vi "Convert From Subpanel Tag.vi"(8 "error in":errorcluster, 11 "subpanel tag":string) -> (0 "error out":errorcluster, 1 "valid?":bool, 2 "subpanel UID":i32, 3 "owning VI name":string)   [LabVIEW 2010, in "NI_SE_Config Front Panel Layout.lvlib"]
uses:
  NI_SE_Config Front Panel Layout.lvlib
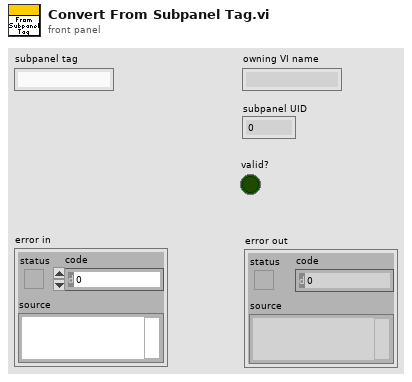
[diagram p1: front panel]
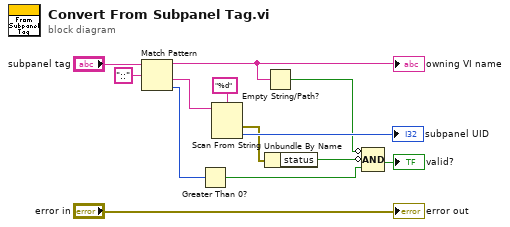
[diagram p0: block diagram]
diagram:
  n1 = Match Pattern(string="subpanel tag", regular expression="::") -> (before substring=w4:string, after substring=w10:string, offset past match=w7:i32)  [unwired: 1 in, 1 out]
  "owning VI name" <- w4
  n2 = Greater Than 0?(x=w7) -> (x > 0?=w6:bool)
  n3 = Scan From String(format string="%d", input string=w10) -> (error out=w3:errorcluster, output 1=→"subpanel UID":i32)  [unwired: 3 in, 2 out]
  n4 = Empty String/Path?(string/path=w4) -> (empty?=w2:bool)
  n5 = Unbundle By Name(w3) -> ("status"=w1:bool)
  n6 = Compound Arithmetic op=AND(invert w2, invert w1, w6) -> (→"valid?":bool)
  "error out" <- "error in"
